vi "Data_Packet_FGV.vi"(0 "Data_Packet In":T1={"Packet"={"Raw Bytes"=[], "Checksum"=FALSE, "Direction"=enum."Transmit", "Processed Bytes"=[], "Node ID"=0, "Packet type"=enum."Connection Management", "Frame Data"=0, "Priority"=enum."LOW", "Frame ID"=0}, "Parameters"=[], "Last Received Time (ms)"=0, "Receive count"=0, "Transmit count"=0, "Transmit interval (ms)"=0, "Last Transmitted Time (ms)"=0, "Receive interval (ms)"=0, "Transmit_Mode"=enum."Disabled", "Transmit Enable"=FALSE, "Cyclic Transmit interval (ms)"=0}, 2 "Symbol File Path":path, 5 "Parameters In":T6[](array[typedef]), 7 "Node ID":u8, 9 "Frame ID":u8, 11 "error in (no error)":errorcluster, 12 "Parameter name":string, 13 "Commands":T9=enum."Load") -> (3 "Node ID output":u8, 4 "Data Packets Out":T1[](array[typedef]), 6 "Parameters out":T6[](array[typedef]), 8 "Data_Packet out":T1={"Packet"={"Raw Bytes"=[], "Checksum"=FALSE, "Direction"=enum."Transmit", "Processed Bytes"=[], "Node ID"=0, "Packet type"=enum."Connection Management", "Frame Data"=0, "Priority"=enum."LOW", "Frame ID"=0}, "Parameters"=[], "Last Received Time (ms)"=0, "Receive count"=0, "Transmit count"=0, "Transmit interval (ms)"=0, "Last Transmitted Time (ms)"=0, "Receive interval (ms)"=0, "Transmit_Mode"=enum."Disabled", "Transmit Enable"=FALSE, "Cyclic Transmit interval (ms)"=0}, 14 "Frame ID output":u8, 15 "error out":errorcluster)   [LabVIEW 2017]
uses:
  Controls/Data Packets/Data_Packet_FGV_Commands.ctl
  Controls/Data Packets/Parameter.ctl
  Controls/Data Packets/Parameter_Data_Type.ctl
  Controls/Data Packets/Data_Packet.ctl
  Controls/Packet/Packet.ctl
  Controls/Packet/Packet_Direction.ctl
  Controls/Packet/Packet_Type.ctl
  Controls/Packet/Packet_Priority.ctl
  Controls/Data Packets/Data_Packet_Transmit_Mode.ctl
panel:
  out "Parameters":T6[](array[typedef])
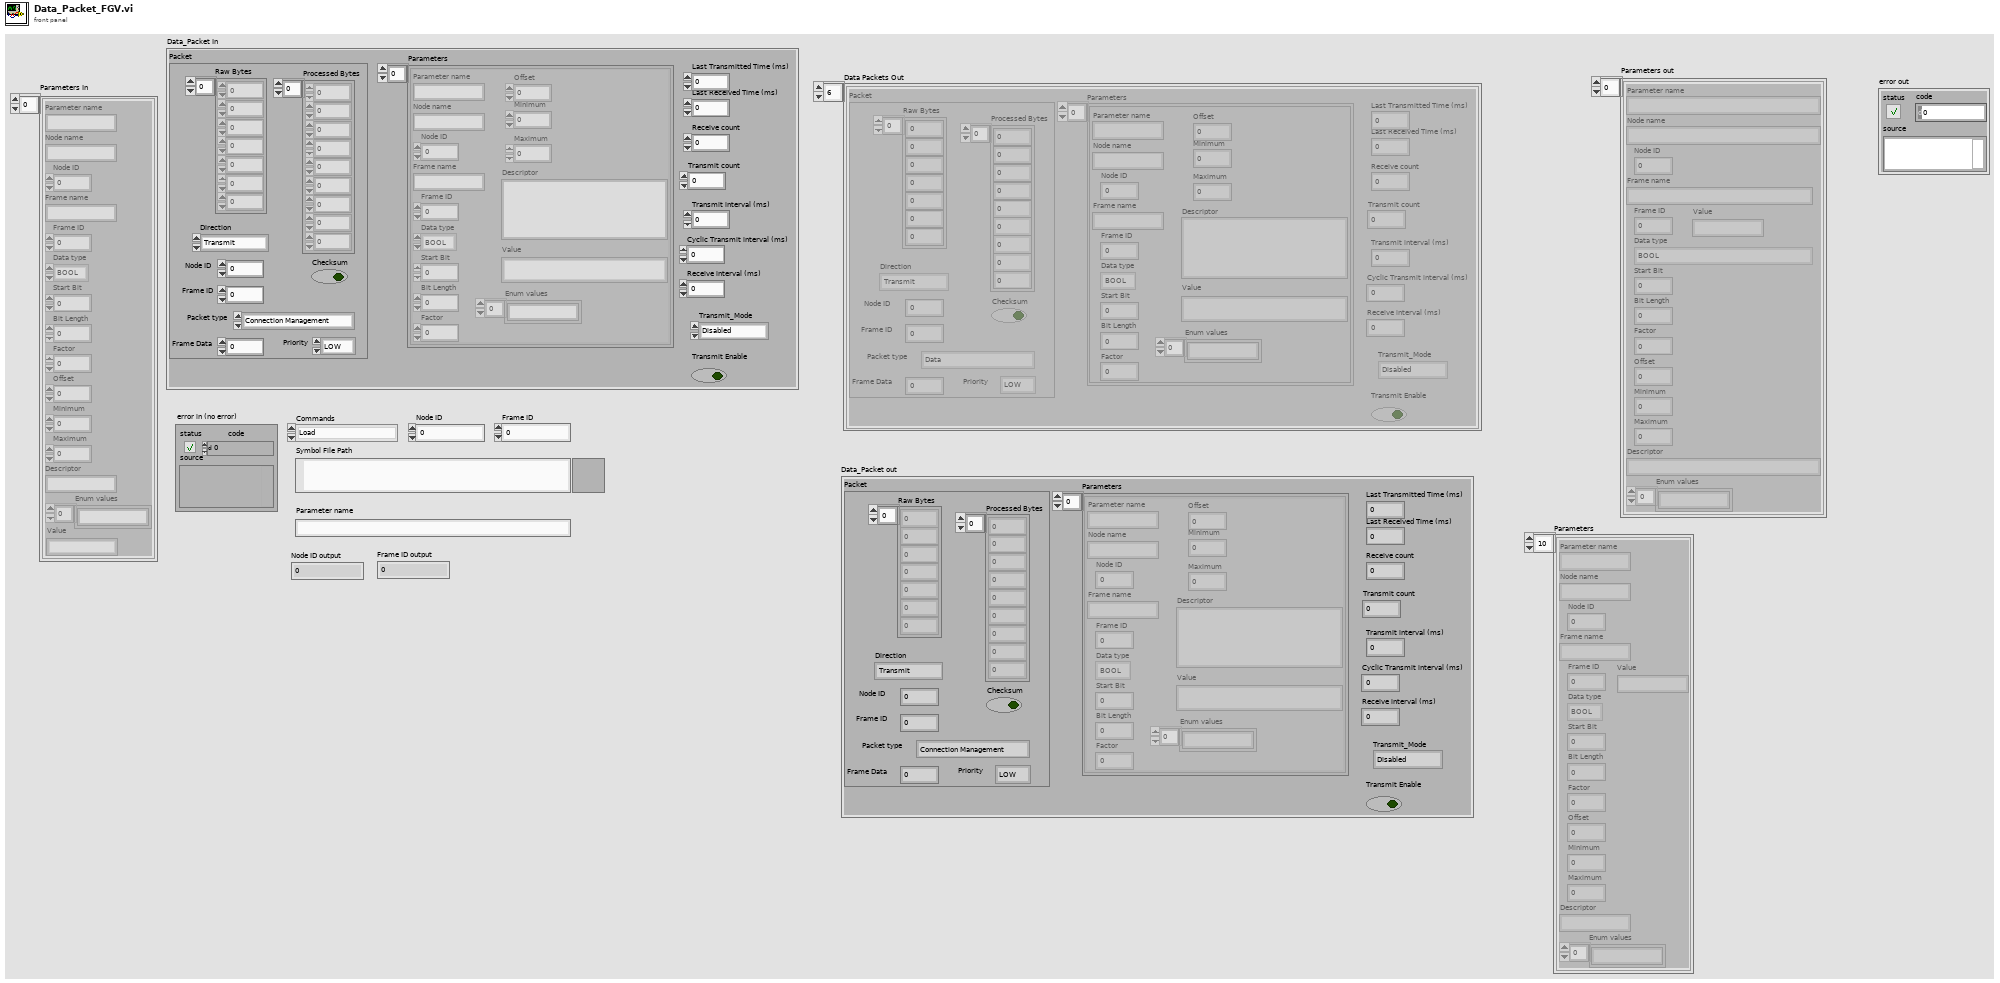
[diagram p1: front panel]
types:
  T1 = typedef "Data_Packet.ctl" = cluster{"Packet":T2, "Parameters":T6[], "Last Received Time (ms)":u64, "Receive count":i32, "Transmit count":i32, "Transmit interval (ms)":u32, "Last Transmitted Time (ms)":u64, "Receive interval (ms)":u32, "Transmit_Mode":T8, "Transmit Enable":bool, "Cyclic Transmit interval (ms)":u32}
  T2 = typedef "Packet.ctl" = cluster{"Raw Bytes":u8[], "Checksum":bool, "Direction":T3, "Processed Bytes":u8[], "Node ID":u8, "Packet type":T4, "Frame Data":u32, "Priority":T5, "Frame ID":u8}
  T3 = typedef "Packet_Direction.ctl" = enum16{"Transmit", "Receive", "Bidirectional"}
  T4 = typedef "Packet_Type.ctl" = enum16{"Data", "Connection Management", "Remote Request", "Error/Status"}
  T5 = typedef "Packet_Priority.ctl" = enum16{"LOW", "HIGH"}
  T6 = typedef "Parameter.ctl" = cluster{"Parameter name":string, "Node name":string, "Node ID":u8, "Frame name":string, "Frame ID":u8, "Data type":T7, "Start Bit":i32, "Bit Length":i32, "Factor":dbl, "Offset":dbl, "Minimum":dbl, "Maximum":dbl, "Descriptor":string, "Enum values":string[], "Value":string}
  T7 = typedef "Parameter_Data_Type.ctl" = enum16{"BOOL", "UNSIGNED", "SIGNED", "FLOAT32", "ENUM"}
  T8 = typedef "Data_Packet_Transmit_Mode.ctl" = enum16{"Disabled", "Single", "Cyclic"}
  T9 = typedef "Data_Packet_FGV_Commands.ctl" = enum16{"Update all parameters from data packets", "Update Packet", "Load", "Read Packet Parameters", "Write Packet Parameters", "Read Packet Parameter", "Write Packet Parameter", "Read Data Packets", "Read Data Packet", "Read Data Packet by Parameter Name", "Get Parameter Node and Frame ID", "Read Data Packet from Node ID and Frame ID"}
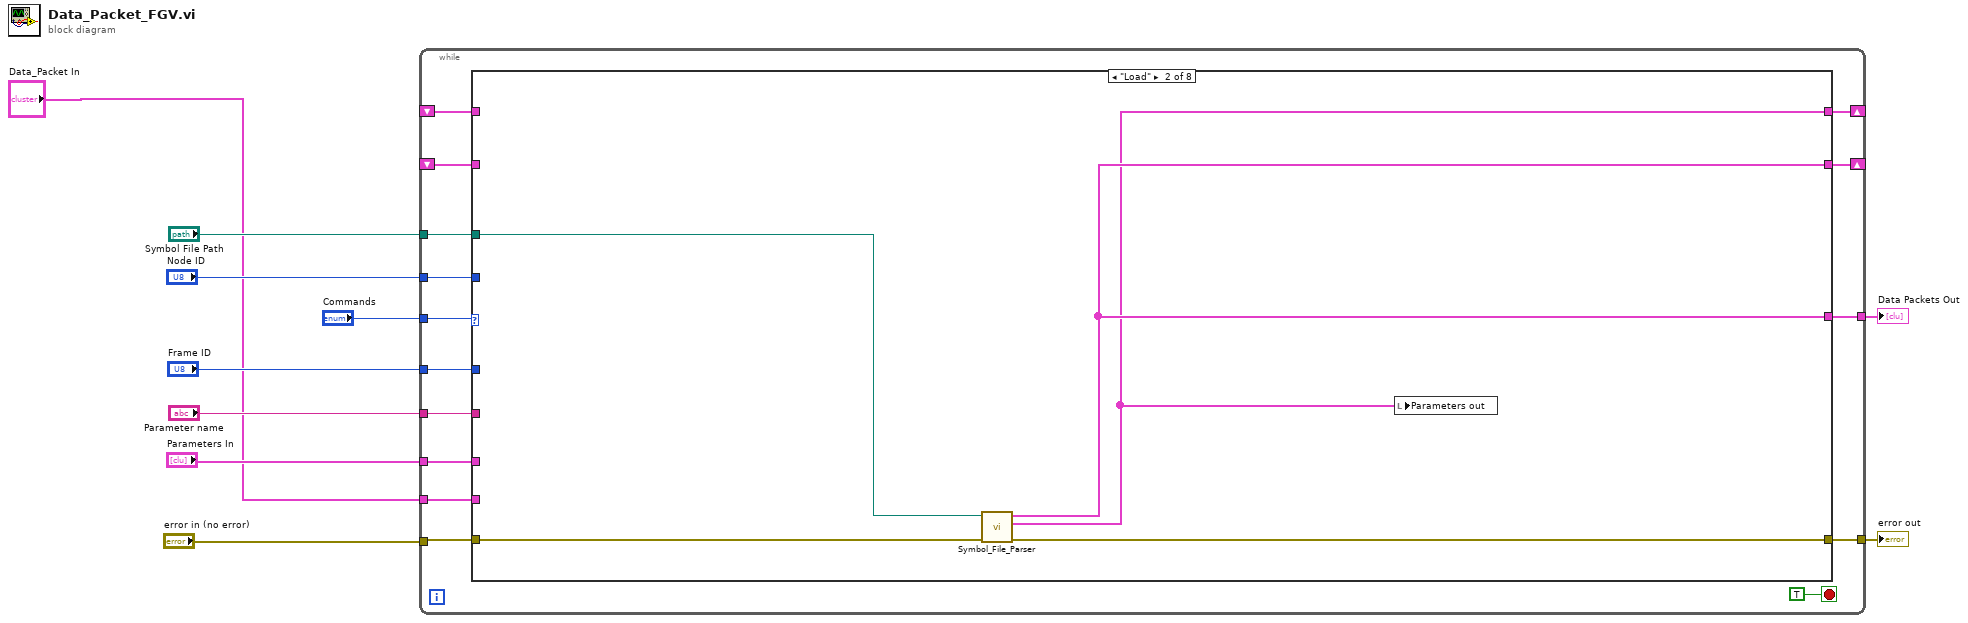
[diagram p0: block diagram]
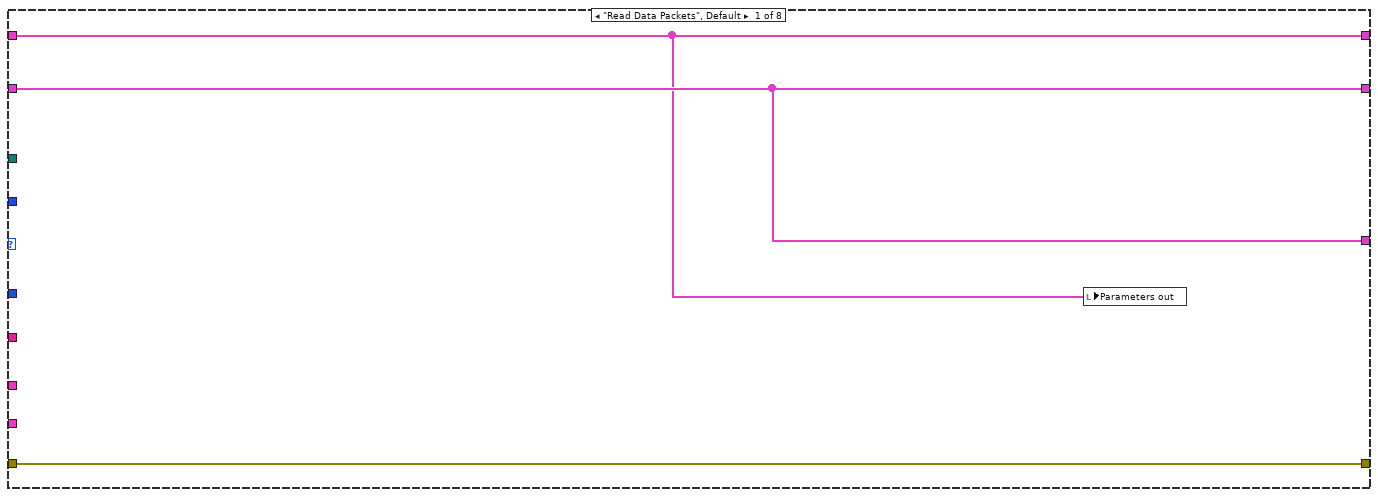
[diagram p2: hidden frame]
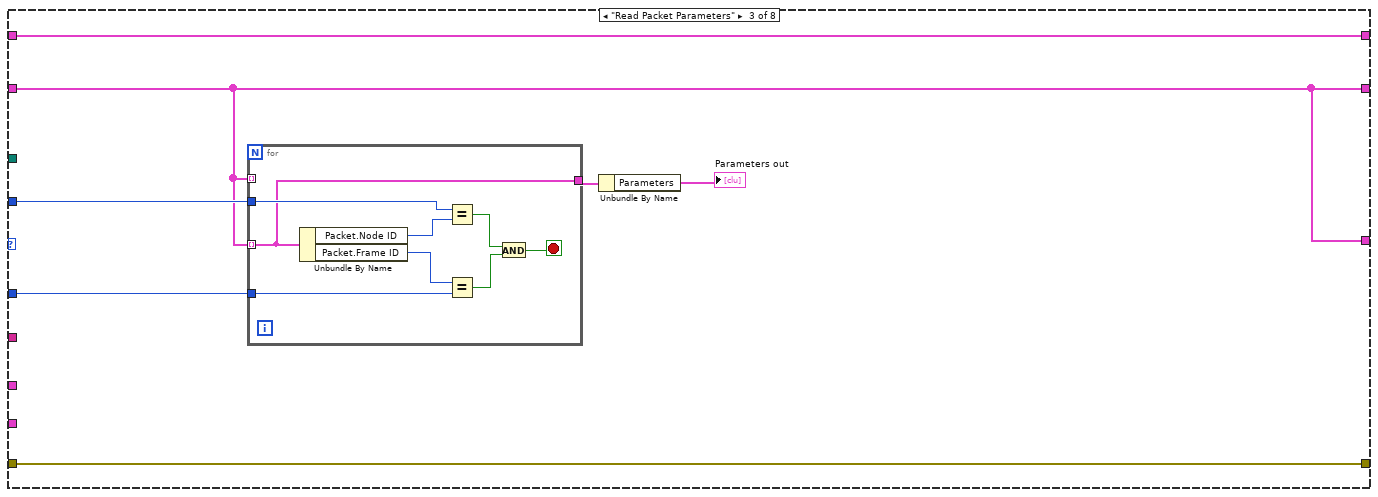
[diagram p3: hidden frame]
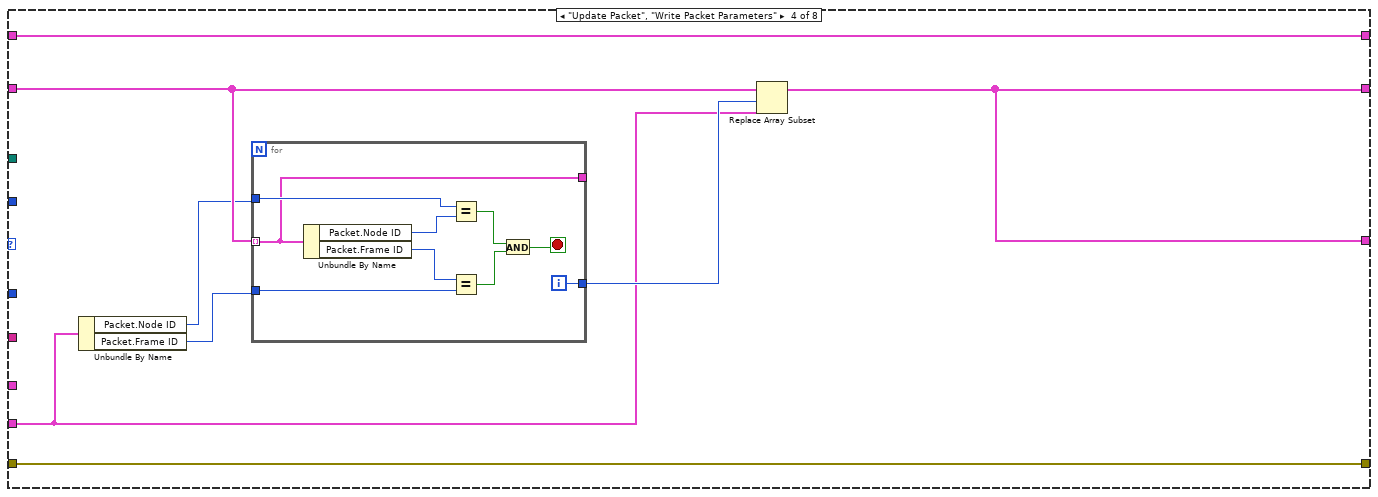
[diagram p4: hidden frame]
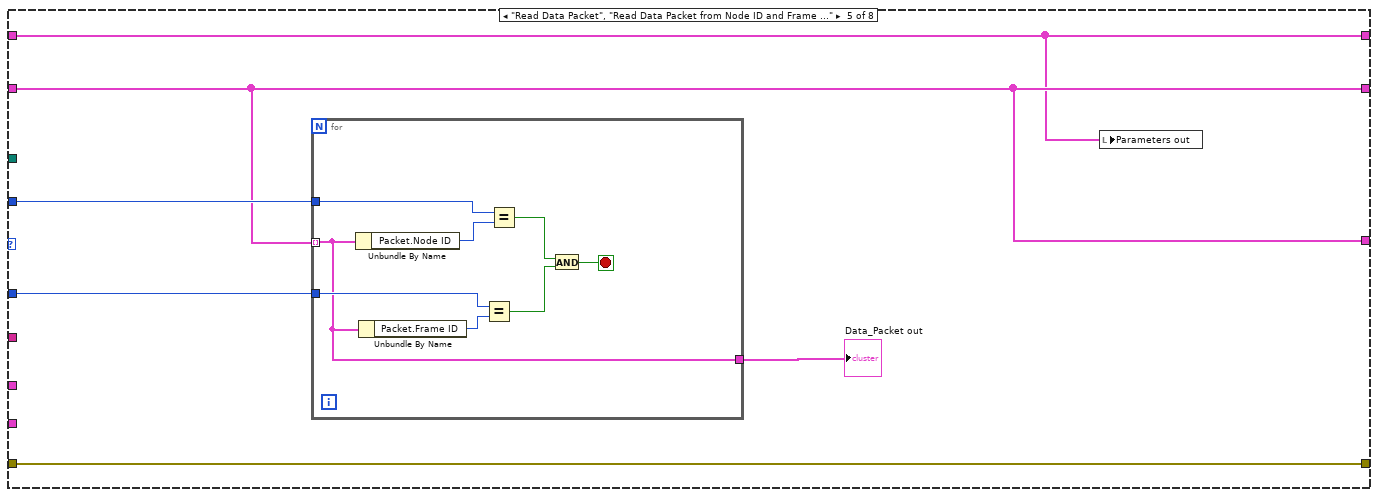
[diagram p5: hidden frame]
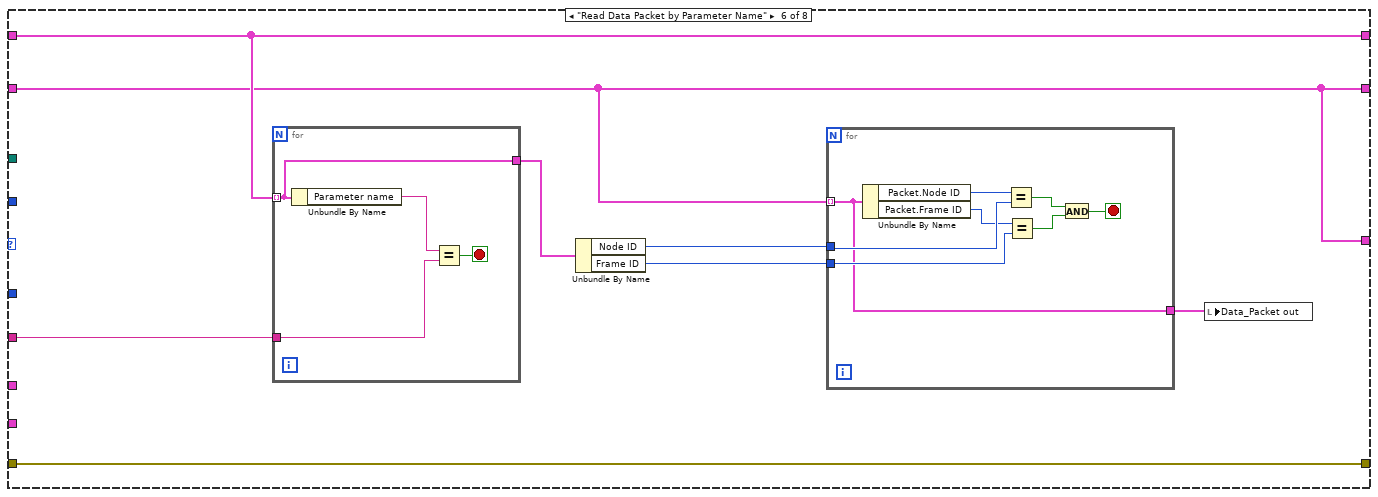
[diagram p6: hidden frame]
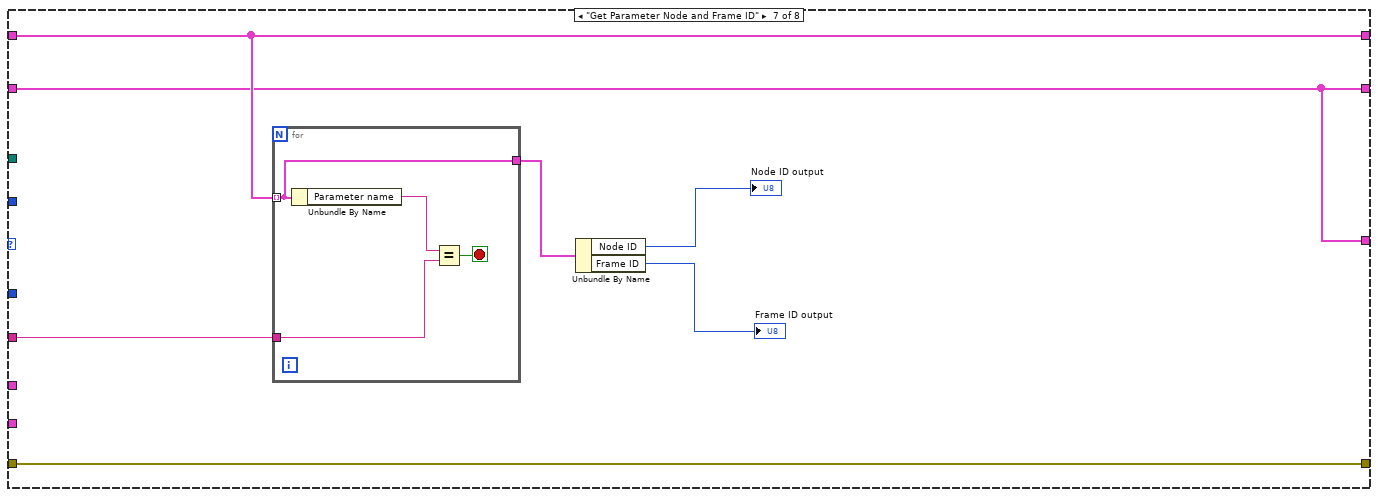
[diagram p7: hidden frame]
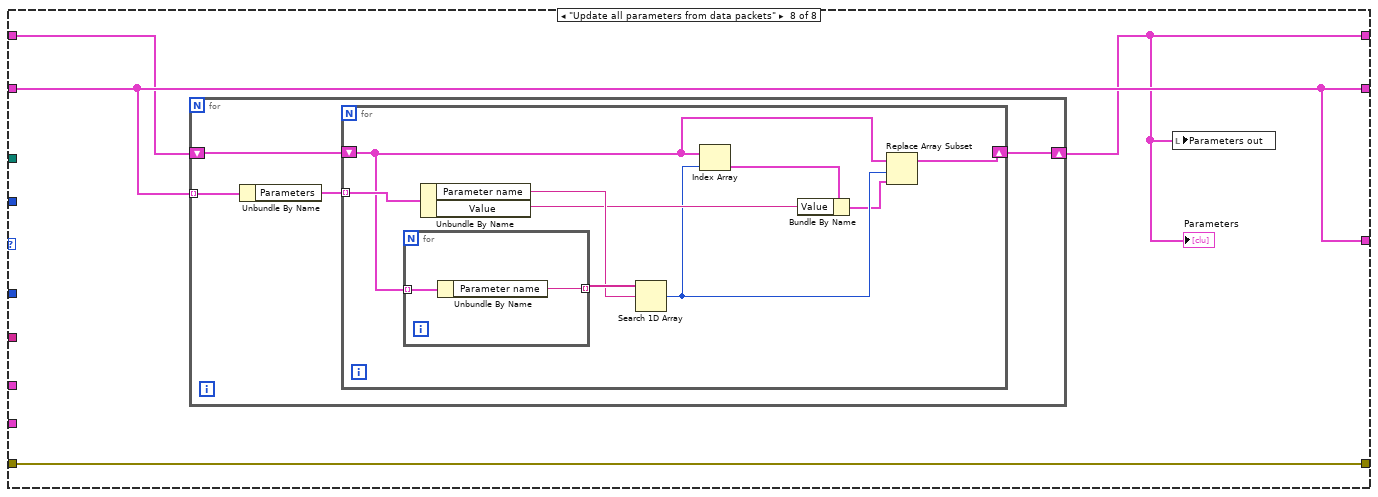
[diagram p8: hidden frame]
diagram:
  n1 = while {
    tunnel: "error in (no error)" -> [w22]
    tunnel: "Commands" -> [w24]
    tunnel: "Symbol File Path" -> [w23]
    shift-right: [w21] -> _
    shift-left: _ -> [w20]
    tunnel: [w19] -> w3
    tunnel: "Node ID" -> [w18]
    tunnel: "Frame ID" -> [w17]
    tunnel: [w16] -> w5
    tunnel: "Parameters In" -> [w15]
    shift-right: [w14] -> _
    shift-left: _ -> [w13]
    tunnel: "Parameter name" -> [w12]
    tunnel: "Data_Packet In" -> [w11]
    stop <- TRUE stop-if-true
    n2 = case shown="\"Load\"" w24 {
      tunnel: w23 -> [_ w32 _ _ _ _ _ _]
      tunnel: w22 -> [w28 w33 w35 w53 w68 w81 w102 w114]
      tunnel: [w27 w30 w38 w54 w69 w84 w103 w113] -> w21
      tunnel: w20 -> [w27 _ w38 w56 w69 w84 w103 w113]
      tunnel: [w28 w31 w35 w53 w68 w81 w102 w114] -> w19
      tunnel: w18 -> [_ _ w40 _ w71 _ _ _]
      tunnel: w17 -> [_ _ w39 _ w70 _ _ _]
      tunnel: [w27 w30 w38 w54 w69 w84 w103 w113] -> w16
      tunnel: w15 -> [_ _ _ _ _ _ _ _]
      tunnel: [w26 w29 w34 w52 w67 w87 w106 w111] -> w14
      tunnel: w13 -> [w26 _ w34 w52 w67 w87 w106 w112]
      tunnel: w12 -> [_ _ _ _ _ w86 w105 _]
      tunnel: w11 -> [_ _ _ w51 _ _ _ _]
      frame "Read Data Packets", Default {
        n3 = local write "Parameters out"(w26) -> ()
      }
      frame "Load" {
        n4 = call "Symbol_File_Parser.vi"("error in (no error)"=w33, "Symbol File Path"=w32) -> ("error out"=w31:errorcluster, "Parameters"=w29:T6[], "Data Packets"=w30:T1[])  [unwired: 7 in]
        n5 = local write "Parameters out"(w29) -> ()
      }
      frame "Read Packet Parameters" {
        n6 = for {
          tunnel: w38 -> [w41] mode=indexing
          tunnel: w40 -> [w47]
          tunnel: w39 -> [w45]
          tunnel: w38 -> [_] mode=indexing
          tunnel: [w41] -> w37
          stop <- w42 stop-if-true
          n7 = Unbundle By Name(w41) -> ("Packet.Node ID"=w48:u8, "Packet.Frame ID"=w46:u8)
          n8 = Equal?(x=w47, y=w48) -> (x = y?=w44:bool)
          n9 = Equal?(x=w46, y=w45) -> (x = y?=w43:bool)
          n10 = And(x=w44, y=w43) -> (x .and. y?=w42:bool)
        }
        n11 = Unbundle By Name(w37) -> ("Parameters"=→"Parameters out":T6[])
      }
      frame "Update Packet", "Write Packet Parameters" {
        n12 = Unbundle By Name(w51) -> ("Packet.Node ID"=w50:u8, "Packet.Frame ID"=w49:u8)
        n13 = for {
          tunnel: w56 -> [w58] mode=indexing
          tunnel: w50 -> [w64]
          tunnel: w49 -> [w62]
          tunnel: [w58] -> _
          tunnel: [w57] -> w55
          i -> [w57]
          stop <- w59 stop-if-true
          n14 = Unbundle By Name(w58) -> ("Packet.Node ID"=w65:u8, "Packet.Frame ID"=w63:u8)
          n15 = Equal?(x=w64, y=w65) -> (x = y?=w61:bool)
          n16 = Equal?(x=w63, y=w62) -> (x = y?=w60:bool)
          n17 = And(x=w61, y=w60) -> (x .and. y?=w59:bool)
        }
        n18 = Replace Array Subset(array=w56, new element=w51, index=w55) -> (w54:T1[])
      }
      frame "Read Data Packet", "Read Data Packet from Node ID and Frame ID" {
        n19 = for {
          tunnel: w69 -> [w72] mode=indexing
          tunnel: w71 -> [w78]
          tunnel: w70 -> [w76]
          tunnel: [w72] -> w66
          stop <- w73 stop-if-true
          n20 = Unbundle By Name(w72) -> ("Packet.Node ID"=w79:u8)
          n21 = Unbundle By Name(w72) -> ("Packet.Frame ID"=w77:u8)
          n22 = Equal?(x=w76, y=w77) -> (x = y?=w74:bool)
          n23 = Equal?(x=w78, y=w79) -> (x = y?=w75:bool)
          n24 = And(x=w75, y=w74) -> (x .and. y?=w73:bool)
        }
        "Data_Packet out" <- w66
        n25 = local write "Parameters out"(w67) -> ()
      }
      frame "Read Data Packet by Parameter Name" {
        n26 = for {
          tunnel: w87 -> [w97] mode=indexing
          tunnel: w86 -> [w98]
          tunnel: [w97] -> w85
          stop <- w96 stop-if-true
          n27 = Unbundle By Name(w97) -> ("Parameter name"=w99:string)
          n28 = Equal?(x=w99, y=w98) -> (x = y?=w96:bool)
        }
        n29 = Unbundle By Name(w85) -> ("Node ID"=w83:u8, "Frame ID"=w82:u8)
        n30 = for {
          tunnel: w84 -> [w88] mode=indexing
          tunnel: w83 -> [w94]
          tunnel: w82 -> [w92]
          tunnel: [w88] -> w80
          stop <- w89 stop-if-true
          n31 = Unbundle By Name(w88) -> ("Packet.Node ID"=w95:u8, "Packet.Frame ID"=w93:u8)
          n32 = Equal?(x=w95, y=w94) -> (x = y?=w91:bool)
          n33 = Equal?(x=w93, y=w92) -> (x = y?=w90:bool)
          n34 = And(x=w91, y=w90) -> (x .and. y?=w89:bool)
        }
        n35 = local write "Data_Packet out"(w80) -> ()
      }
      frame "Get Parameter Node and Frame ID" {
        n36 = for {
          tunnel: w106 -> [w108] mode=indexing
          tunnel: w105 -> [w109]
          tunnel: [w108] -> w104
          stop <- w107 stop-if-true
          n37 = Unbundle By Name(w108) -> ("Parameter name"=w110:string)
          n38 = Equal?(x=w110, y=w109) -> (x = y?=w107:bool)
        }
        n39 = Unbundle By Name(w104) -> ("Node ID"=→"Node ID output":u8, "Frame ID"=→"Frame ID output":u8)
      }
      frame "Update all parameters from data packets" {
        n40 = for {
          tunnel: w113 -> [w118] mode=indexing
          shift-right: [w115] -> w111
          shift-left: w112 -> [w117]
          n41 = Unbundle By Name(w118) -> ("Parameters"=w116:T6[])
          n42 = for {
            shift-right: [w119] -> w115
            shift-left: w117 -> [w122]
            tunnel: w116 -> [w126] mode=indexing
            n43 = for {
              tunnel: w122 -> [w129] mode=indexing
              tunnel: [w128] -> w127 mode=indexing
              n44 = Unbundle By Name(w129) -> ("Parameter name"=w128:string)
            }
            n45 = Unbundle By Name(w126) -> ("Parameter name"=w125:string, "Value"=w123:string)
            n46 = Search 1D Array(1D array=w127, element=w125) -> (index of element=w121:i32)  [unwired: 1 in]
            n47 = Index Array(array=w122, index=w121) -> (element=w124:T6)
            n48 = Bundle By Name(cluster=w124, "Value"=w123) -> (w120:T6)
            n49 = Replace Array Subset(array=w122, new element=w120, index=w121) -> (w119:T6[])
          }
        }
        "Parameters" <- w111
        n50 = local write "Parameters out"(w111) -> ()
      }
    }
  }
  "Data Packets Out" <- w5
  "error out" <- w3
